vi "Bounds.vi"(1 "XRef":refnum<vi>, 2 "State In":T2) -> (0 "Bounds":cluster{"Width":T1, "Height":T1})   [LabVIEW 2018, in "Unindex and Unbundle.xnode"]
doc: "This ability VI is used to tell LabVIEW your current bounds. If you want to update your bounds, you must inform LabVIEW through the UpdateImageAndBounds reply of another ability VI. If you change your bounds, you will also probably want to update your image.\n\nDefault behavior: None.\n\nThis ability does not provide UI and OS messages are not handled."
uses:
  Unindex and Unbundle.xnode
  State.ctl
  <vilib>/XNodeSupport/XNodeInt.ctl
  <vilib>/XNodeSupport/NI_XNodeSupport.lvlib
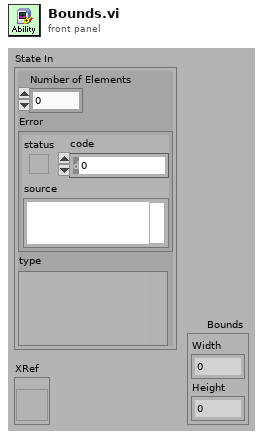
[diagram p1: front panel]
types:
  T1 = typedef "NI_XNodeSupport.lvlib/XNodeInt.ctl" = i32
  T2 = typedef "Unindex and Unbundle.xnode/State.ctl" = cluster{"Number of Elements":i32, "Error":errorcluster, "type":variant}
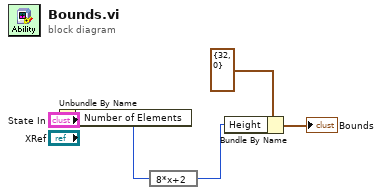
[diagram p0: block diagram]
diagram:
  n1 = Unbundle By Name("State In") -> ("Number of Elements"=w2:i32)
  n2 = expression code="8*x+2"(w2) -> (w1:i32)
  n3 = Bundle By Name(cluster=cluster{"Width":T1, "Height":T1} {"Width"=32, "Height"=0} ("Bounds"), "Height"=w1) -> (→"Bounds":cluster{"Width":T1, "Height":T1})
